vi "Move Into Control.vi"() -> ()   [LabVIEW 2023]
doc: "Demonstrates the Move method in VI Scripting to programmatically move an object from one location to another, where the destination is a container object."
uses:
  <vilib>/Utility/miscctls.llb/LVPositionTypeDef.ctl
panel:
  in  "Move Me - Numeric":string="Move Me - Numeric"
  in  "Destination Cluster":string="Destination Cluster"
  # "Overview: Demonstrates the Move method in VI Scripting to programmatically move an object from one location to another.\nInstructions:\n1. Open the front panels of Test - Moving Objects Source.vi and Test - Moving Objects Target.vi.\n2. Run this VI. The \"Move Me - Numeric\" control will be copied from the source VI into the \"Destination Cluster\" in the target VI.\n\nNote: When moving an object from one VI to another, the operation results in a copy, since the original object is preserved. When moving an object to a different location in the same VI, it will not be a copy operation unless the Duplicate? parameter of the Move method is set to TRUE."
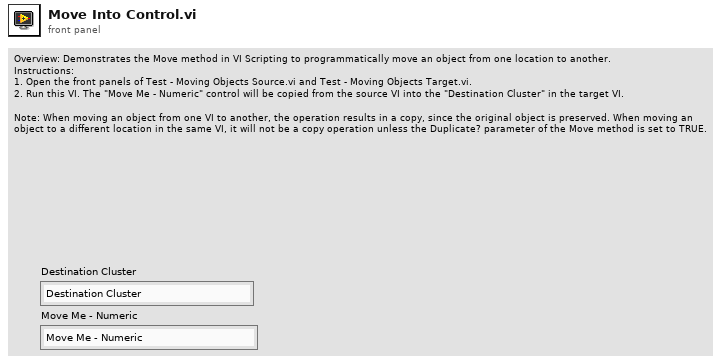
[diagram p1: front panel]
types:
  T1 = typedef "LVPositionTypeDef.ctl" = cluster{"Left":i32, "Top":i32}
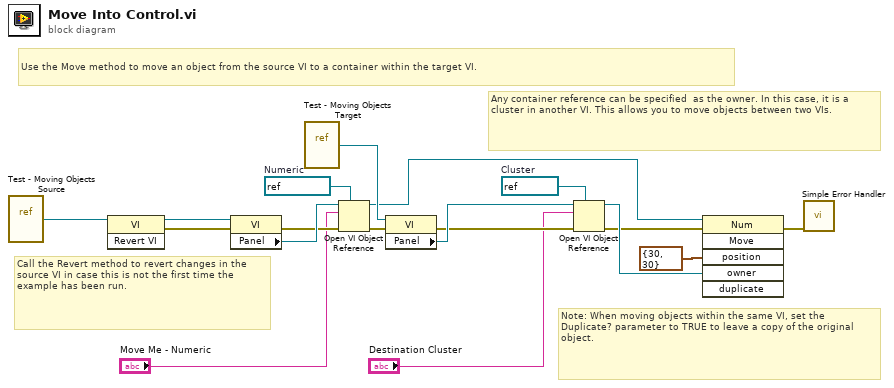
[diagram p0: block diagram]
diagram:
  w3 = refnum<vi> refnum  # Cluster
  w5 = refnum<vi> refnum  # Numeric
  # "Note: When moving objects within the same VI, set the Duplicate? parameter to TRUE to leave a copy of the original object."
  # "Any container reference can be specified  as the owner. In this case, it is a cluster in another VI. This allows you to move objects between two VIs."
  # "Call the Revert method to revert changes in the source VI in case this is not the first time the example has been run."
  # "Use the Move method to move an object from the source VI to a container within the target VI."
  n1 = vi-ref "Test - Moving Objects Source.vi"() -> (w17:refnum<vi>)
  n2 = invoke class="VI" method="Revert VI"(reference=w17) -> (reference out=w16:refnum<vi>, error out=w15:errorcluster)  [unwired: 2 in, 1 out]
  n3 = property class="VI"(reference=w16, error in=w15) -> (error out=w9:errorcluster, "Panel"=w13:refnum<vi>)  [unwired: 1 out]
  n4 = vi-ref "Test - Moving Objects Target.vi"() -> (w18:refnum<vi>)
  n5 = Open VI Object Reference(7:w5, 8:w9, 10:"Move Me - Numeric", 11:w13) -> (0:w8:errorcluster, 3:w1:refnum<vi>)
  n6 = property class="VI"(reference=w18, error in=w8) -> (error out=w7:errorcluster, "Panel"=w11:refnum<vi>)  [unwired: 1 out]
  n7 = Open VI Object Reference(7:w3, 8:w7, 10:"Destination Cluster", 11:w11) -> (0:w6:errorcluster, 3:w10:refnum<vi>)
  n8 = invoke class="Num" method="Move"(reference=w1, error in=w6, "position"=T1 {"Left"=30, "Top"=30}, "owner"=w10) -> (error out=w14:errorcluster)  [unwired: 2 in, 5 out]
  n9 = call <vilib>:"Simple Error Handler.vi"("error in (no error)"=w14) -> ()  [unwired: 4 in, 5 out]
